vi "Set Execution Unit Inline.vi"(5 "Inline Rx UDP":bool caption="Inline Rx UDP Execution", 7 "Inline Tx UDP":bool caption="Inline Tx UDP Execution", 8 "error in":errorcluster, 9 "Inline Inline Rx Monitor":bool caption="Inline Rx Monitor  Execution", 10 "Inline Tx Generic Execution":bool, 11 "custom device ref":T1 format="%.0x") -> (0 "error out":errorcluster, 3 "custom device ref out":T1 format="%.0x")   [LabVIEW 2020, in "AIM ARINC 664 Scripting.lvlib"]
uses:
  AIM ARINC 664 Scripting.lvlib
  <vilib>/NI VeriStand/Custom Device API/Custom Device Item Ref.ctl
  Constants.vi
  <vilib>/NI VeriStand/Custom Device API/Set Item Property (Boolean).vi
  <vilib>/NI VeriStand/Custom Device API/Custom Device API.lvlib
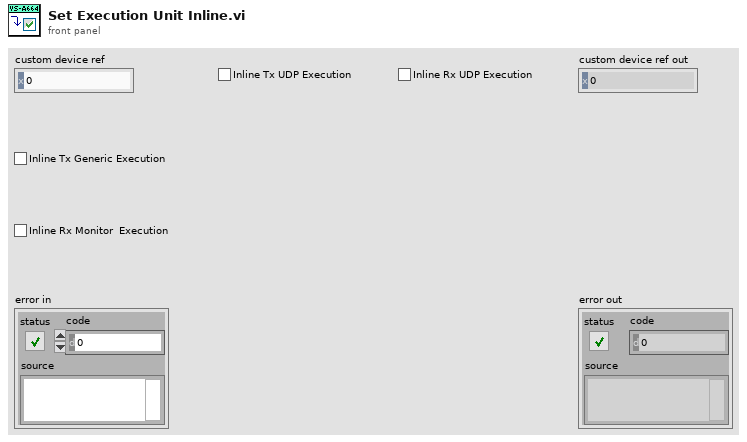
[diagram p1: front panel]
types:
  T1 = typedef "Custom Device API.lvlib/Custom Device Item Ref.ctl" = u64
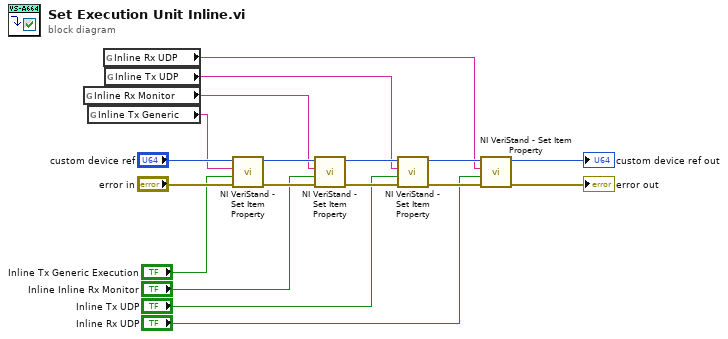
[diagram p0: block diagram]
diagram:
  n1 = global read "Constants.vi" "Inline Rx Monitor"() -> (w3:string)
  n2 = global read "Constants.vi" "Inline Tx Generic"() -> (w4:string)
  n3 = global read "Constants.vi" "Inline Rx UDP"() -> (w1:string)
  n4 = global read "Constants.vi" "Inline Tx UDP"() -> (w2:string)
  n5 = call-poly <vilib>:"NI VeriStand - Set Item Property.vi"("error in (no error)"="error in", "Value"="Inline Tx Generic Execution", "Property Name"=w4, "Item Ref in"="custom device ref") -> ("error out"=w12:errorcluster, "Item Ref out"=w17:T1)  [unwired: 5 in, 1 out]
  n6 = call-poly <vilib>:"NI VeriStand - Set Item Property.vi"("error in (no error)"=w12, "Value"="Inline Inline Rx Monitor", "Property Name"=w3, "Item Ref in"=w17) -> ("error out"=w11:errorcluster, "Item Ref out"=w16:T1)  [unwired: 5 in, 1 out]
  n7 = call-poly <vilib>:"NI VeriStand - Set Item Property.vi"("error in (no error)"=w11, "Value"="Inline Tx UDP", "Property Name"=w2, "Item Ref in"=w16) -> ("error out"=w10:errorcluster, "Item Ref out"=w15:T1)  [unwired: 5 in, 1 out]
  n8 = call-poly <vilib>:"NI VeriStand - Set Item Property.vi"("error in (no error)"=w10, "Value"="Inline Rx UDP", "Property Name"=w1, "Item Ref in"=w15) -> ("error out"=→"error out":errorcluster, "Item Ref out"=→"custom device ref out":T1)  [unwired: 5 in, 1 out]
